vi "PAN_SetTimeout.vi"(8 "error in (no error)":errorcluster, 9 "action":T1(ring), 10 "timeout":i32, 11 "Command":string) -> (0 "error out":errorcluster, 2 "obsID":string)   [LabVIEW 2016]
uses:
  Modules/DBSHAND/private/vis/DatabaseHand_Element_Get(string).vi
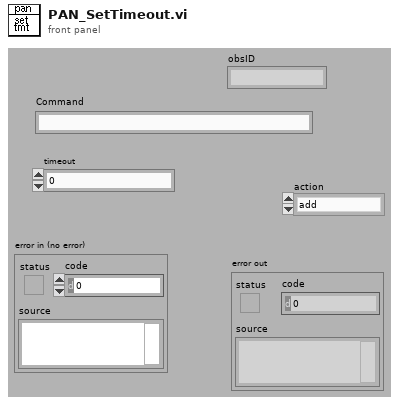
[diagram p1: front panel]
types:
  T1 = enum16{"add", "delete", "clean", "shutdown", "hold", "continue", "modify"}
  T2 = typedef "DatabaseHand_RefNum.ctl" = refnum<vi>
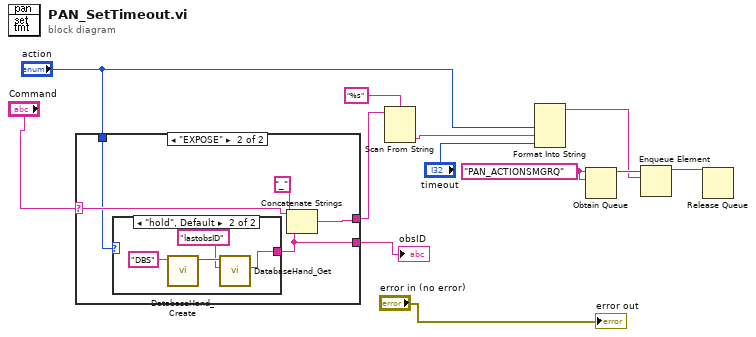
[diagram p0: block diagram]
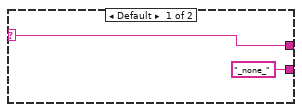
[diagram p2: hidden frame]
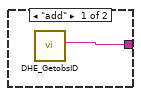
[diagram p3: hidden frame]
diagram:
  w12 = "PAN_ACTIONSMGRQ" ("name (unnamed)")
  n1 = case shown="\"EXPOSE\"" "Command" {
    selector: "Command" -> [w14 w19]
    tunnel: [w14 w18] -> w3
    tunnel: ["_none_" ("obsID") w17] -> w2
    tunnel: "action" -> [_ w15]
    frame Default {
    }
    frame "EXPOSE" {
      n2 = case shown="\"hold\", Default" w15 {
        tunnel: [w20 w21] -> w17
        frame "add" {
          n3 = call "DHE_GetobsID.vi"() -> ("obsID"=w20:string)  [unwired: 1 in, 10 out]
        }
        frame "hold", Default {
          n4 = call "DatabaseHand_Create.vi"("Name"="DBS") -> ("Database RefNum out"=w24:T2)  [unwired: 1 in, 9 out]
          n5 = call-poly "DatabaseHand_Get.vi"("name"="lastobsID", "Database RefNum in"=w24) -> ("value"=w21:string)  [unwired: 3 in, 6 out]
        }
      }
      n6 = Concatenate Strings(w19, "_" ("string"), w17) -> (w18:string)
    }
  }
  "obsID" <- w2
  n7 = Scan From String(format string="%s", input string=w3) -> (output 1=w6:string)  [unwired: 2 in, 4 out]
  n8 = Format Into String("action", w6, "timeout") -> (resulting string=w10:string)  [unwired: 3 in, 1 out]
  n9 = Obtain Queue(name (unnamed)=w12, element data type=w12) -> (queue out=w11:refnum<queue>)  [unwired: 3 in, 2 out]
  n10 = Enqueue Element(queue=w11, element=w10) -> (queue out=w9:refnum<queue>)  [unwired: 1 in, 3 out]
  n11 = Release Queue(queue=w9) -> ()  [unwired: 1 in, 4 out]
  "error out" <- "error in (no error)"
